vi "Zedver_v3_ComCluster.vi"() -> ()   [LabVIEW 2011]
uses:
  Control 1.ctl
panel:
  in  "input cluster":T2={"Petición"="1", "Longitud datos"=0.0, "Longitudes"=[], "Datos"=[]}
  out "String del cluster 5":string
  out "String del cluster 4":string
  out "String del cluster 3":string
  out "String del cluster 2":string
  out "String del cluster":string
  in  "PROCE CSV":path
  in  "HISTO CSV":path
  in  "RAW CSV":path
  in  "Datos procesado":dbl[](array[numeric])
  in  "Datos histograma":dbl[](array[numeric])
  in  "Datos RAW":dbl[](array[numeric])
  in  "Procesado":bool
  out "Bytes procesado":dbl
  out "Bytes histograma":dbl
  out "Bytes RAW":dbl
  in  "Histograma":bool
  in  "RAW":bool
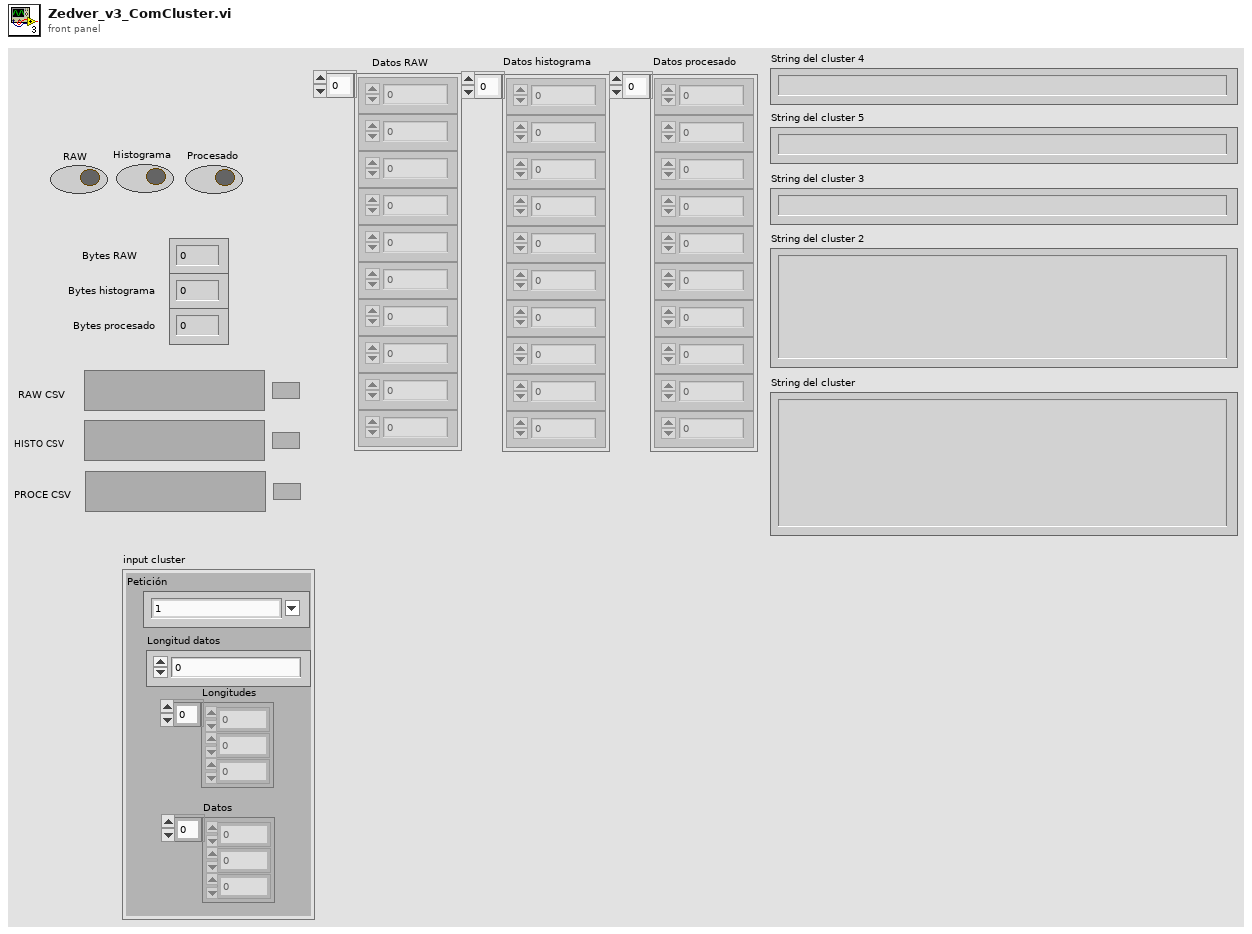
[diagram p1: front panel]
types:
  T1 = typedef "Control 1.ctl" = string
  T2 = cluster{"Petición":T1, "Longitud datos":dbl, "Longitudes":dbl[], "Datos":dbl[]}
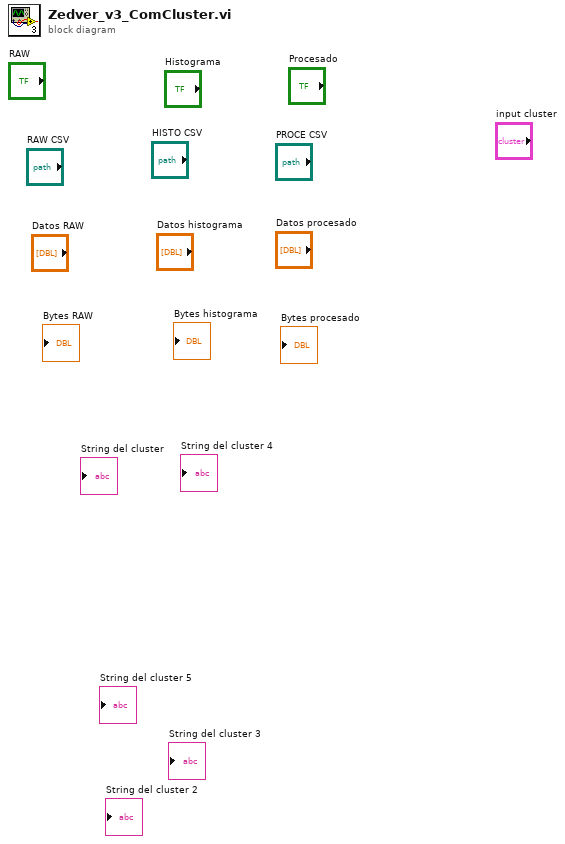
[diagram p0: block diagram]
diagram:
